vi "VisionOpen.vi"(8 "error in (no error)":errorcluster, 11 "Vision in":refnum<class "Vision.lvclass">) -> (0 "error out":errorcluster, 3 "Vision out":refnum<class "Vision.lvclass">)   [LabVIEW 2018, in "Vision.lvclass"]
uses:
  Vision.lvclass
  Vision.lvclass/Vision.ctl
  X-Pixel.vi
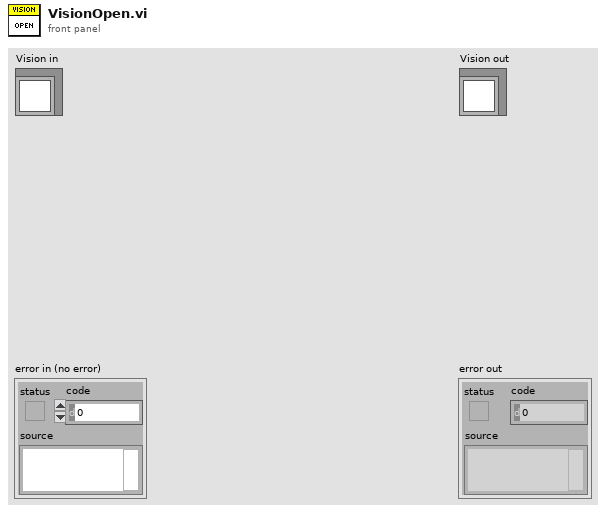
[diagram p1: front panel]
types:
  T1 = cluster{"proportional gain (Kc)":dbl, "integral time (Ti, min)":dbl, "derivative time (Td, min)":dbl}
  T2 = cluster{"LinearAcceleration X":dbl, "LinearAcceleration Y":dbl, "LinearAcceleration Z":dbl}
  T3 = cluster{"Yaw":dbl, "Roll":dbl, "Pitch":dbl, "Heading":dbl, "Fused Heading":dbl}
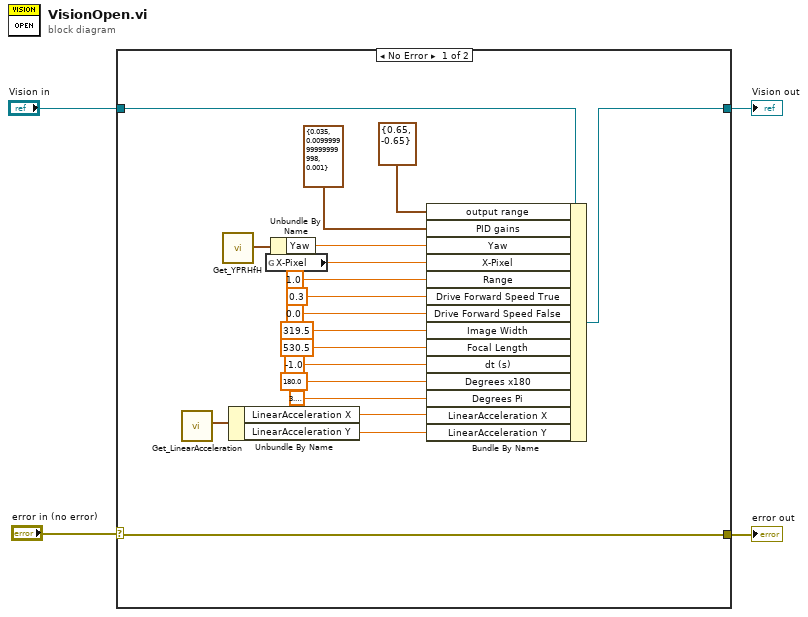
[diagram p0: block diagram]
diagram:
  n1 = case shown="No Error" "error in (no error)" {
    selector: "error in (no error)" -> [w23 w25]
    tunnel: [w23 w25] -> w3
    tunnel: [w20 w24] -> w1
    tunnel: "Vision in" -> [w21 w24]
    frame No Error {
      n2 = call <vilib>:"Get_LinearAcceleration.vi"() -> ("Linear Acceleration"=w7:T2)  [unwired: 11 in]
      n3 = call <vilib>:"Get_YPRHfH.vi"() -> ("YRPHfH"=w22:T3)  [unwired: 11 in]
      n4 = Unbundle By Name(w7) -> ("LinearAcceleration X"=w6:dbl, "LinearAcceleration Y"=w5:dbl)
      n5 = global read "X-Pixel.vi" "X-Pixel"() -> (w18:dbl)
      n6 = Unbundle By Name(w22) -> ("Yaw"=w19:dbl)
      n7 = Bundle By Name(cluster=w21, "output range"=cluster{"output high":dbl, "output low":dbl} {"output high"=0.65, "output low"=-0.65}, "PID gains"=T1 {"proportional gain (Kc)"=0.035, "integral time (Ti, min)"=0.009999999999999998, "derivative time (Td, min)"=0.001}, "Yaw"=w19, "X-Pixel"=w18, "Range"=1.0, "Drive Forward Speed True"=0.3, "Drive Forward Speed False"=0.0, "Image Width"=319.5, "Focal Length"=530.5, "dt (s)"=-1.0, "Degrees x180"=180.0, "Degrees Pi"=3.141592653589793, "LinearAcceleration X"=w6, "LinearAcceleration Y"=w5) -> (w20:refnum<class "Vision.lvclass">)
    }
    frame Error {
    }
  }
  "error out" <- w3
  "Vision out" <- w1
